vi "sleep_detection.vi"(0 "Deprivation\nparameters":T1={"Frame Row"=0, "Kstd"=40.0, "# Images for\nsleep detection"=10, "Kmean"=1.5, "Start time of sleep detection (images):"=1000, 0, "Length (images)"=3600, "# TTL"=10000, "by x images after first detection"=0, "Between TTL pulses"=0, "\nby x detections"=9, "# Total immobility\n detections"=0.0, "max # adjacent\nTTL"=0.0, "TTL x start\ntime deprivation\n"=0.0, "Max #\nadjacent TTL"=10000, " Ca2+\nmode"=0} {"?" items=["1", "2", "3", "4"]; "Frame Row" items=["1", "2", "3", "4"]}, 2 "Input \nparameters":T3={"Frame rate (ms)"=2000, "Worm strain"="N2", "# Images"=0, "State"=enum."Image acquisition", "Time elapsed"=0.0, "Max_num_runs"=100000, "#TTL"=0, "Time of start TTL"=100000, "ImSub Value"=0, "Time of last TTL"=0, "Number of Columns"=2, "Number of Rows"=2, "# AdjacentTTL"=0, "Start sleep detection"="", "Sleep Detection"=FALSE, "# Sleep detections"=0, "Time of first sleep detection"=0, "Time max # adjacent TTL"=0, "Image t-1"=[], "Image t"=[]} {"Number of Rows" items=["1"=1, "2"=2, "3"=3, "4"=4]; "Number of Columns" items=["1"=1, "2"=2, "3"=3, "4"=4]}, 4 "Manual sleep detection":bool) -> (9 "Output \nparameters":T4={"Frame rate (ms)"=2000, "Worm strain"="N2", "Time t"=0, "State"=enum."Image acquisition", "Time elapsed"=0.0, "Max_num_runs"=100000, "#TTL"=0, "Time of start TTL"=100000, "ImSub Value"=0, "Time of last TTL"=0, "Number of Columns"=2, "Number of Rows"=2, "# AdjacentTTL"=0, "Start sleep detection"="", "Sleep Detection"=FALSE, "# Sleep detections"=0, "Time of first sleep detection"=0, "Time max # adjacent TTL"=0, "Image t-1"=[], "Image t"=[]} {"Number of Rows" items=["1"=1, "2"=2, "3"=3, "4"=4]; "Number of Columns" items=["1"=1, "2"=2, "3"=3, "4"=4]})   [LabVIEW 2011]
uses:
  state.ctl
  Action-Init-Update-Get.ctl
panel:
  # "Sleep deprivation settings"
  # "Select deprivation animal"
  # "Row"
  # "Column"
  # "Sleep detection parameters"
  # "Sleep deprivation parameters"
  # "Delay deprivation start:"
  # "Pause deprivation (images):"
  # "Stop deprivation after:"
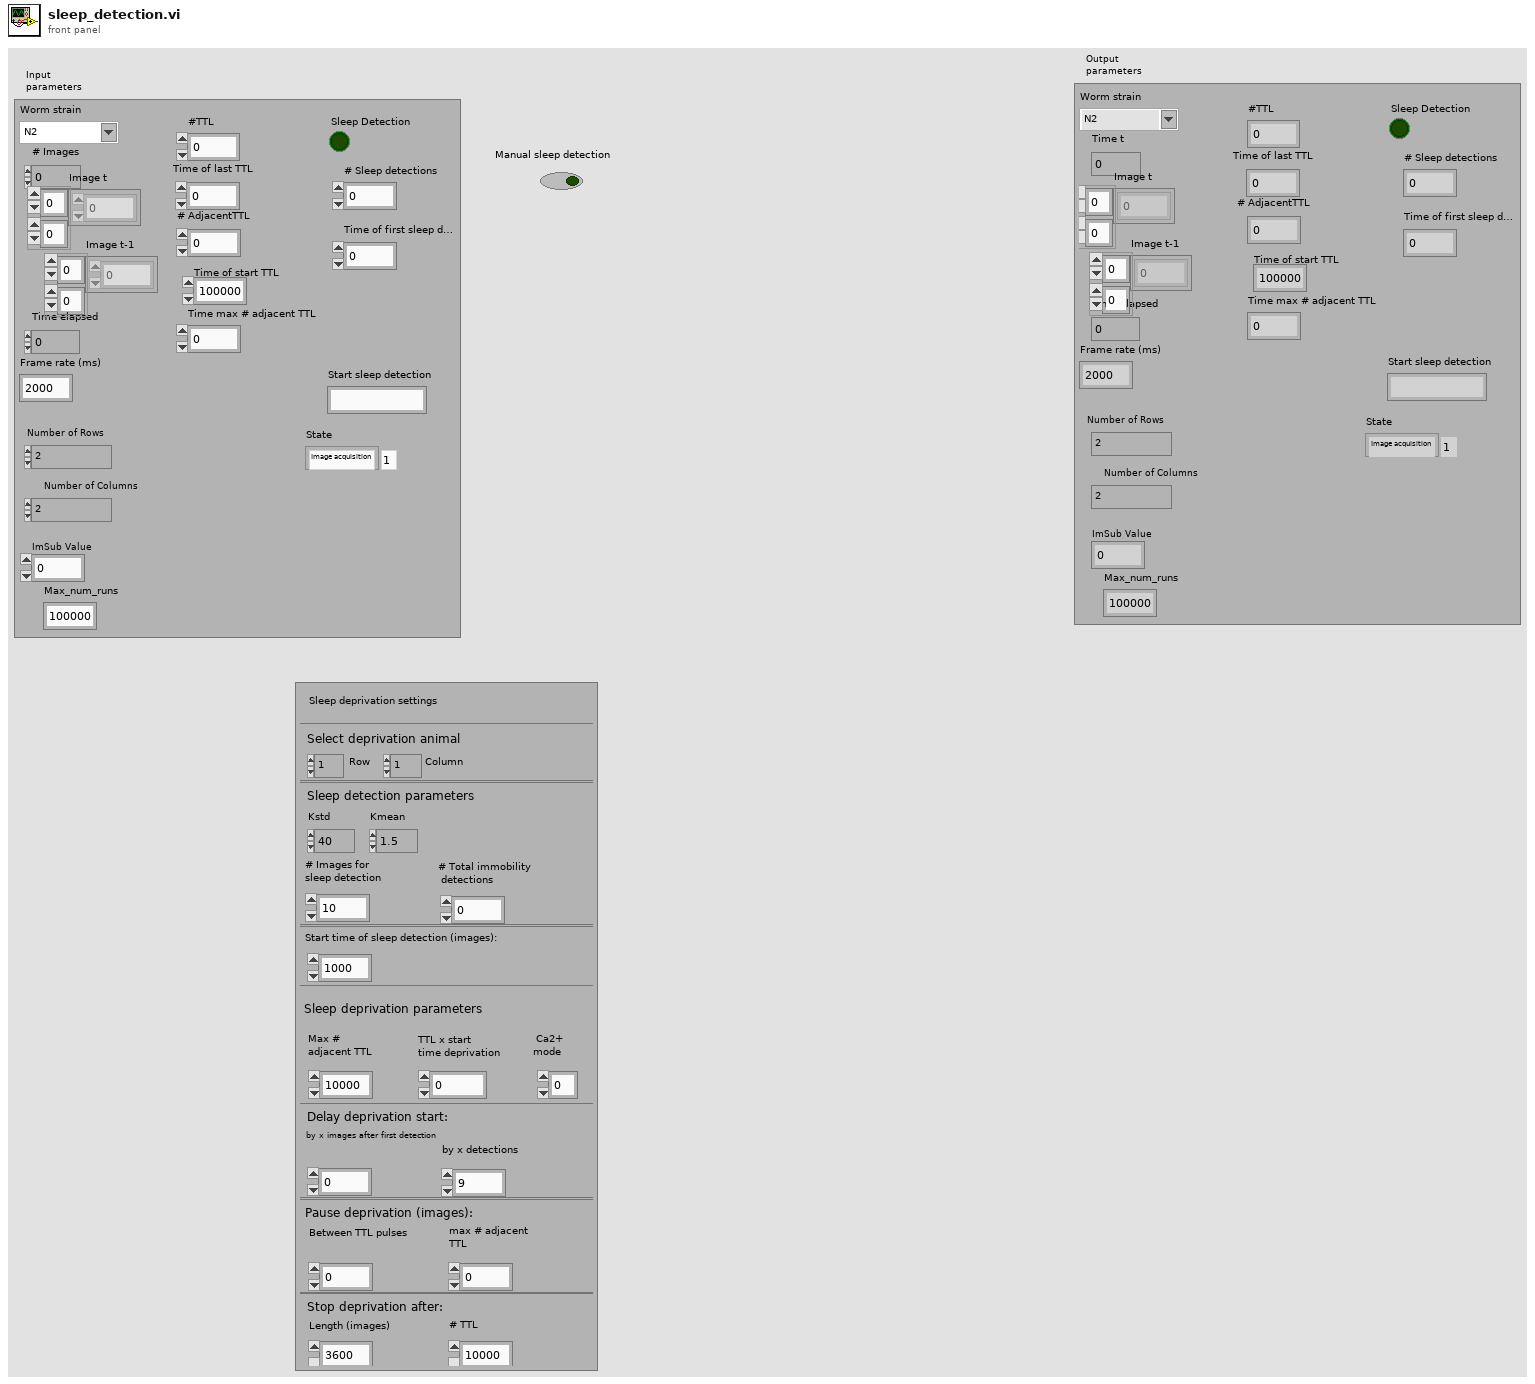
[diagram p1: front panel]
types:
  T1 = cluster{"Frame Row":u32, "Kstd":dbl, "# Images for\nsleep detection":i32, "Kmean":dbl, "Start time of sleep detection (images):":i32, u32, "Length (images)":i32, "# TTL":i32, "by x images after first detection":i32, "Between TTL pulses":i32, "\nby x detections":i32, "# Total immobility\n detections":dbl, "max # adjacent\nTTL":dbl, "TTL x start\ntime deprivation\n":dbl, "Max #\nadjacent TTL":i32, " Ca2+\nmode":i32}
  T2 = typedef "state.ctl" = enum16{"Initialize measurement", "Image acquisition", "Image processing", "Sleep detection", "Control TTL protocol ", "Sleep deprivation", "Update image & exit condition", "Wait "}
  T3 = cluster{"Frame rate (ms)":u32, "Worm strain":string, "# Images":i32, "State":T2, "Time elapsed":dbl, "Max_num_runs":i32, "#TTL":i32, "Time of start TTL":i32, "ImSub Value":i32, "Time of last TTL":i32, "Number of Columns":u32, "Number of Rows":u32, "# AdjacentTTL":i32, "Start sleep detection":string, "Sleep Detection":bool, "# Sleep detections":i32, "Time of first sleep detection":i32, "Time max # adjacent TTL":i32, "Image t-1":i32[][], "Image t":i32[][]}
  T4 = cluster{"Frame rate (ms)":u32, "Worm strain":string, "Time t":i32, "State":T2, "Time elapsed":dbl, "Max_num_runs":i32, "#TTL":i32, "Time of start TTL":i32, "ImSub Value":i32, "Time of last TTL":i32, "Number of Columns":u32, "Number of Rows":u32, "# AdjacentTTL":i32, "Start sleep detection":string, "Sleep Detection":bool, "# Sleep detections":i32, "Time of first sleep detection":i32, "Time max # adjacent TTL":i32, "Image t-1":i32[][], "Image t":i32[][]}
  T5 = typedef "Action-Init-Update-Get.ctl" = enum16{"Initialize", "Update", "Get"}
  T6 = cluster{"Frame rate (ms)":u32, "Worm strain":string, "Time t":i32, "State":T2, "Time elapsed":dbl, "Max_num_runs":i32, "#TTL":i32, "SD start reference":i32, "ImSub Value":i32, "Time of last TTL":i32, "Number of Columns":u32, "Number of Rows":u32, "# AdjacentTTL":i32, "Start sleep detection":string, "Sleep Detection":bool, "# Sleep detections":i32, "Time of first sleep detection":i32, "Time max # adjacent TTL":i32, "Image t-1":i32[][], "Image t":i32[][]}
  T7 = cluster{"Frame rate (ms)":u32, "Worm strain":string, "Time t":i32, "State":T2, "Time elapsed":dbl, "Max_num_runs":i32, "#TTL":i32, "Time of start TTL":i32, "ImSub Value":i32, "Time of last TTL":i32, "Number of Columns":u32, "Number of Rows":u32, "# AdjacentTTL":i32, "Sleep deprivation status":string, "Sleep Detection":bool, "# Sleep detections":i32, "Time of first sleep detection":i32, "Time max # adjacent TTL":i32, "Image t-1":i32[][], "Image t":i32[][]}
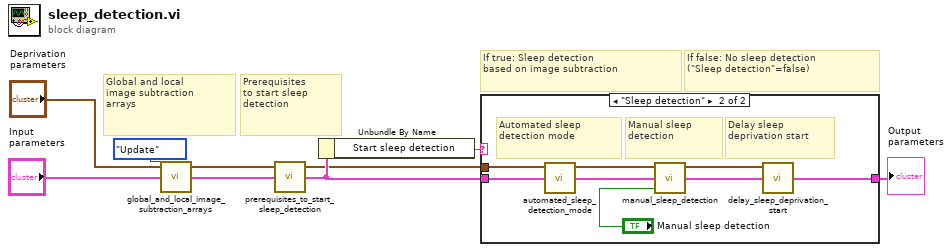
[diagram p0: block diagram]
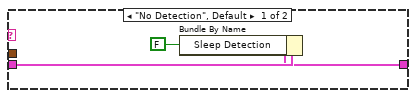
[diagram p2: hidden frame]
diagram:
  # "Global and local\nimage subtraction\narrays"
  # "Prerequisites \nto start sleep\ndetection"
  # "If false: No sleep detection\n(\"Sleep detection\"=false)"
  # "If true: Sleep detection\nbased on image subtraction"
  n1 = call "global_and_local_image_subtraction_arrays.vi"("Input \nparameters"="Input \nparameters", "Deprivation\nparameters"="Deprivation\nparameters", "State"=Action-Init-Update-Get."Update" ("Action")) -> ()  [unwired: 8 in, 1 out]
  n2 = call "prerequisites_to_start_sleep_detection.vi"("Input \nparameters"="Input \nparameters", "Deprivation\nparameters"="Deprivation\nparameters") -> ("Output \nparameters"=w5:T6)  [unwired: 4 in]
  n3 = Unbundle By Name(w5) -> ("Start sleep detection"=w6:string)
  n4 = case shown="\"Sleep detection\"" w6 {
    tunnel: w5 -> [w9 w11]
    tunnel: [w7 w14] -> w1
    tunnel: "Deprivation\nparameters" -> [_ w10]
    frame "No Detection", Default {
      n5 = Bundle By Name(cluster=w9, "Sleep Detection"=FALSE) -> (w7:T6)
    }
    frame "Sleep detection" {
      # "Delay sleep\ndeprivation start"
      # "Automated sleep\ndetection mode"
      # "Manual sleep\ndetection"
      n6 = call "automated_sleep_detection_mode.vi"("Input \nparameters"=w11, "Deprivation\nparameters"=w10) -> ("Output \nparameters"=w13:T7)  [unwired: 4 in]
      n7 = call "manual_sleep_detection.vi"("Input \nparameters"=w13, "Manual sleep detection"="Manual sleep detection") -> ("Output \nParameters"=w12:T7)  [unwired: 9 in]
      n8 = call "delay_sleep_deprivation_start.vi"("Input \nparameters"=w12, "Deprivation\nparameters"=w10) -> ("Output \nparameters"=w14:T7)  [unwired: 1 in]
    }
  }
  "Output \nparameters" <- w1
